vi "grapher.vi"(0 "Eventnum refnum":refnum<vi>, 5 "Frequency refnum":refnum<vi>, 7 "Stop signaller":refnum<class "Signaller.lvclass">, 9 "Polarization refnum":refnum<vi>, 11 "Rate refnum":refnum<vi>) -> ()   [LabVIEW 2018]
uses:
  Motor controller/Signaller/Signaller.lvclass
panel:
  in  "Focus range":dbl=0.1 min=0.001 step=0.1 format="%.3g"
  in  "Focus on current":bool
  in  "Scale for negative":bool
  in  "Scale for positive":bool
  in  "Autoscale polarization":bool=TRUE
  in  "Min polarization":dbl step=0.1 format="%.3g"
  in  "Max polarization":dbl=1.0 step=0.1 format="%.3g"
  in  "Add 1 hour":bool
  in  "1 hour":bool
  in  "30 minutes":bool
  in  "10 minutes":bool
  in  "5 minutes":bool
  in  "1 minute":bool
  in  "Time scale (min)":i64=1 min=1 step=1
  in  "Data output file":path
  out "Data points":i32
  out "Polarization vs frequency":cluster{dbl, dbl}[](graph)
  out "Rate vs time":cluster{"Value":i64, "Value":dbl}[](graph)
  out "Frequency vs time":cluster{"Value":i64, "Value":dbl}[](graph)
  out "Polarization vs time":cluster{i64, dbl}[](graph)
  out "Rate":dbl
  out "Polarization":dbl
  out "Frequency":dbl
  out "Eventnum":i64
  # "Advanced controls"
  # "Graph polarization scale"
  # "Graph time scale"
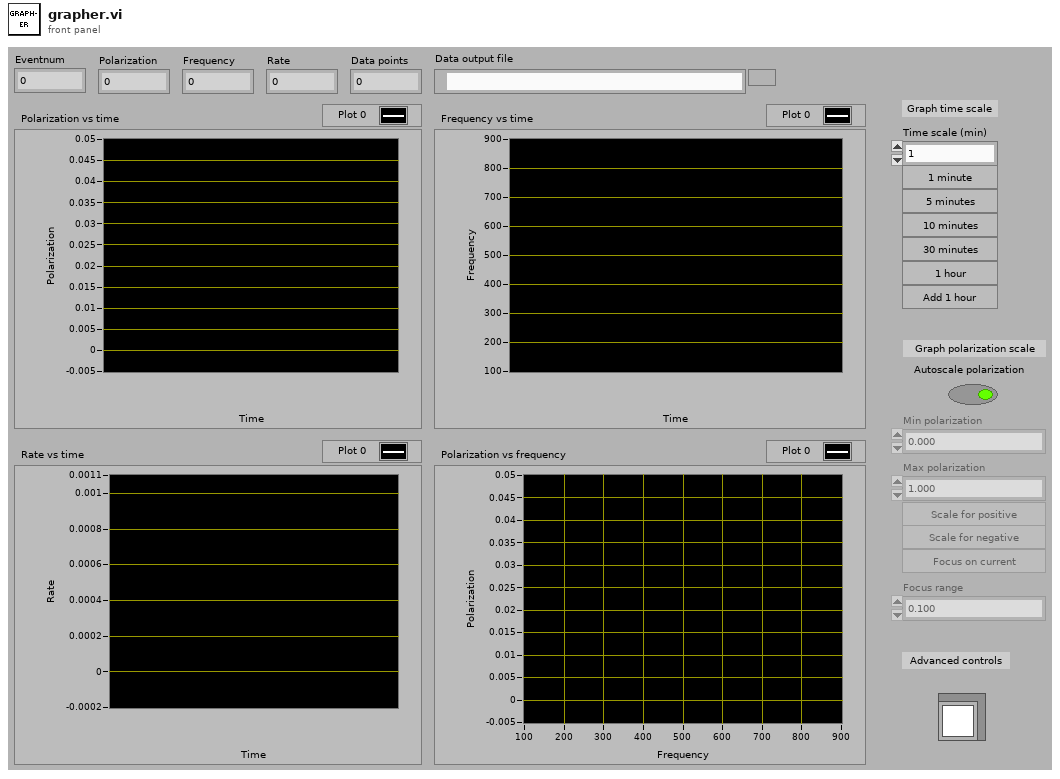
[diagram p1: front panel]
types:
  T1 = typedef "LVRangeTypeDef.ctl" = cluster{"Minimum":dbl, "Maximum":dbl, "Increment":dbl, "Minor Increment":dbl, "Start":dbl}
  T2 = enum8{"Enabled", "Disabled", "Disabled and Grayed Out"}
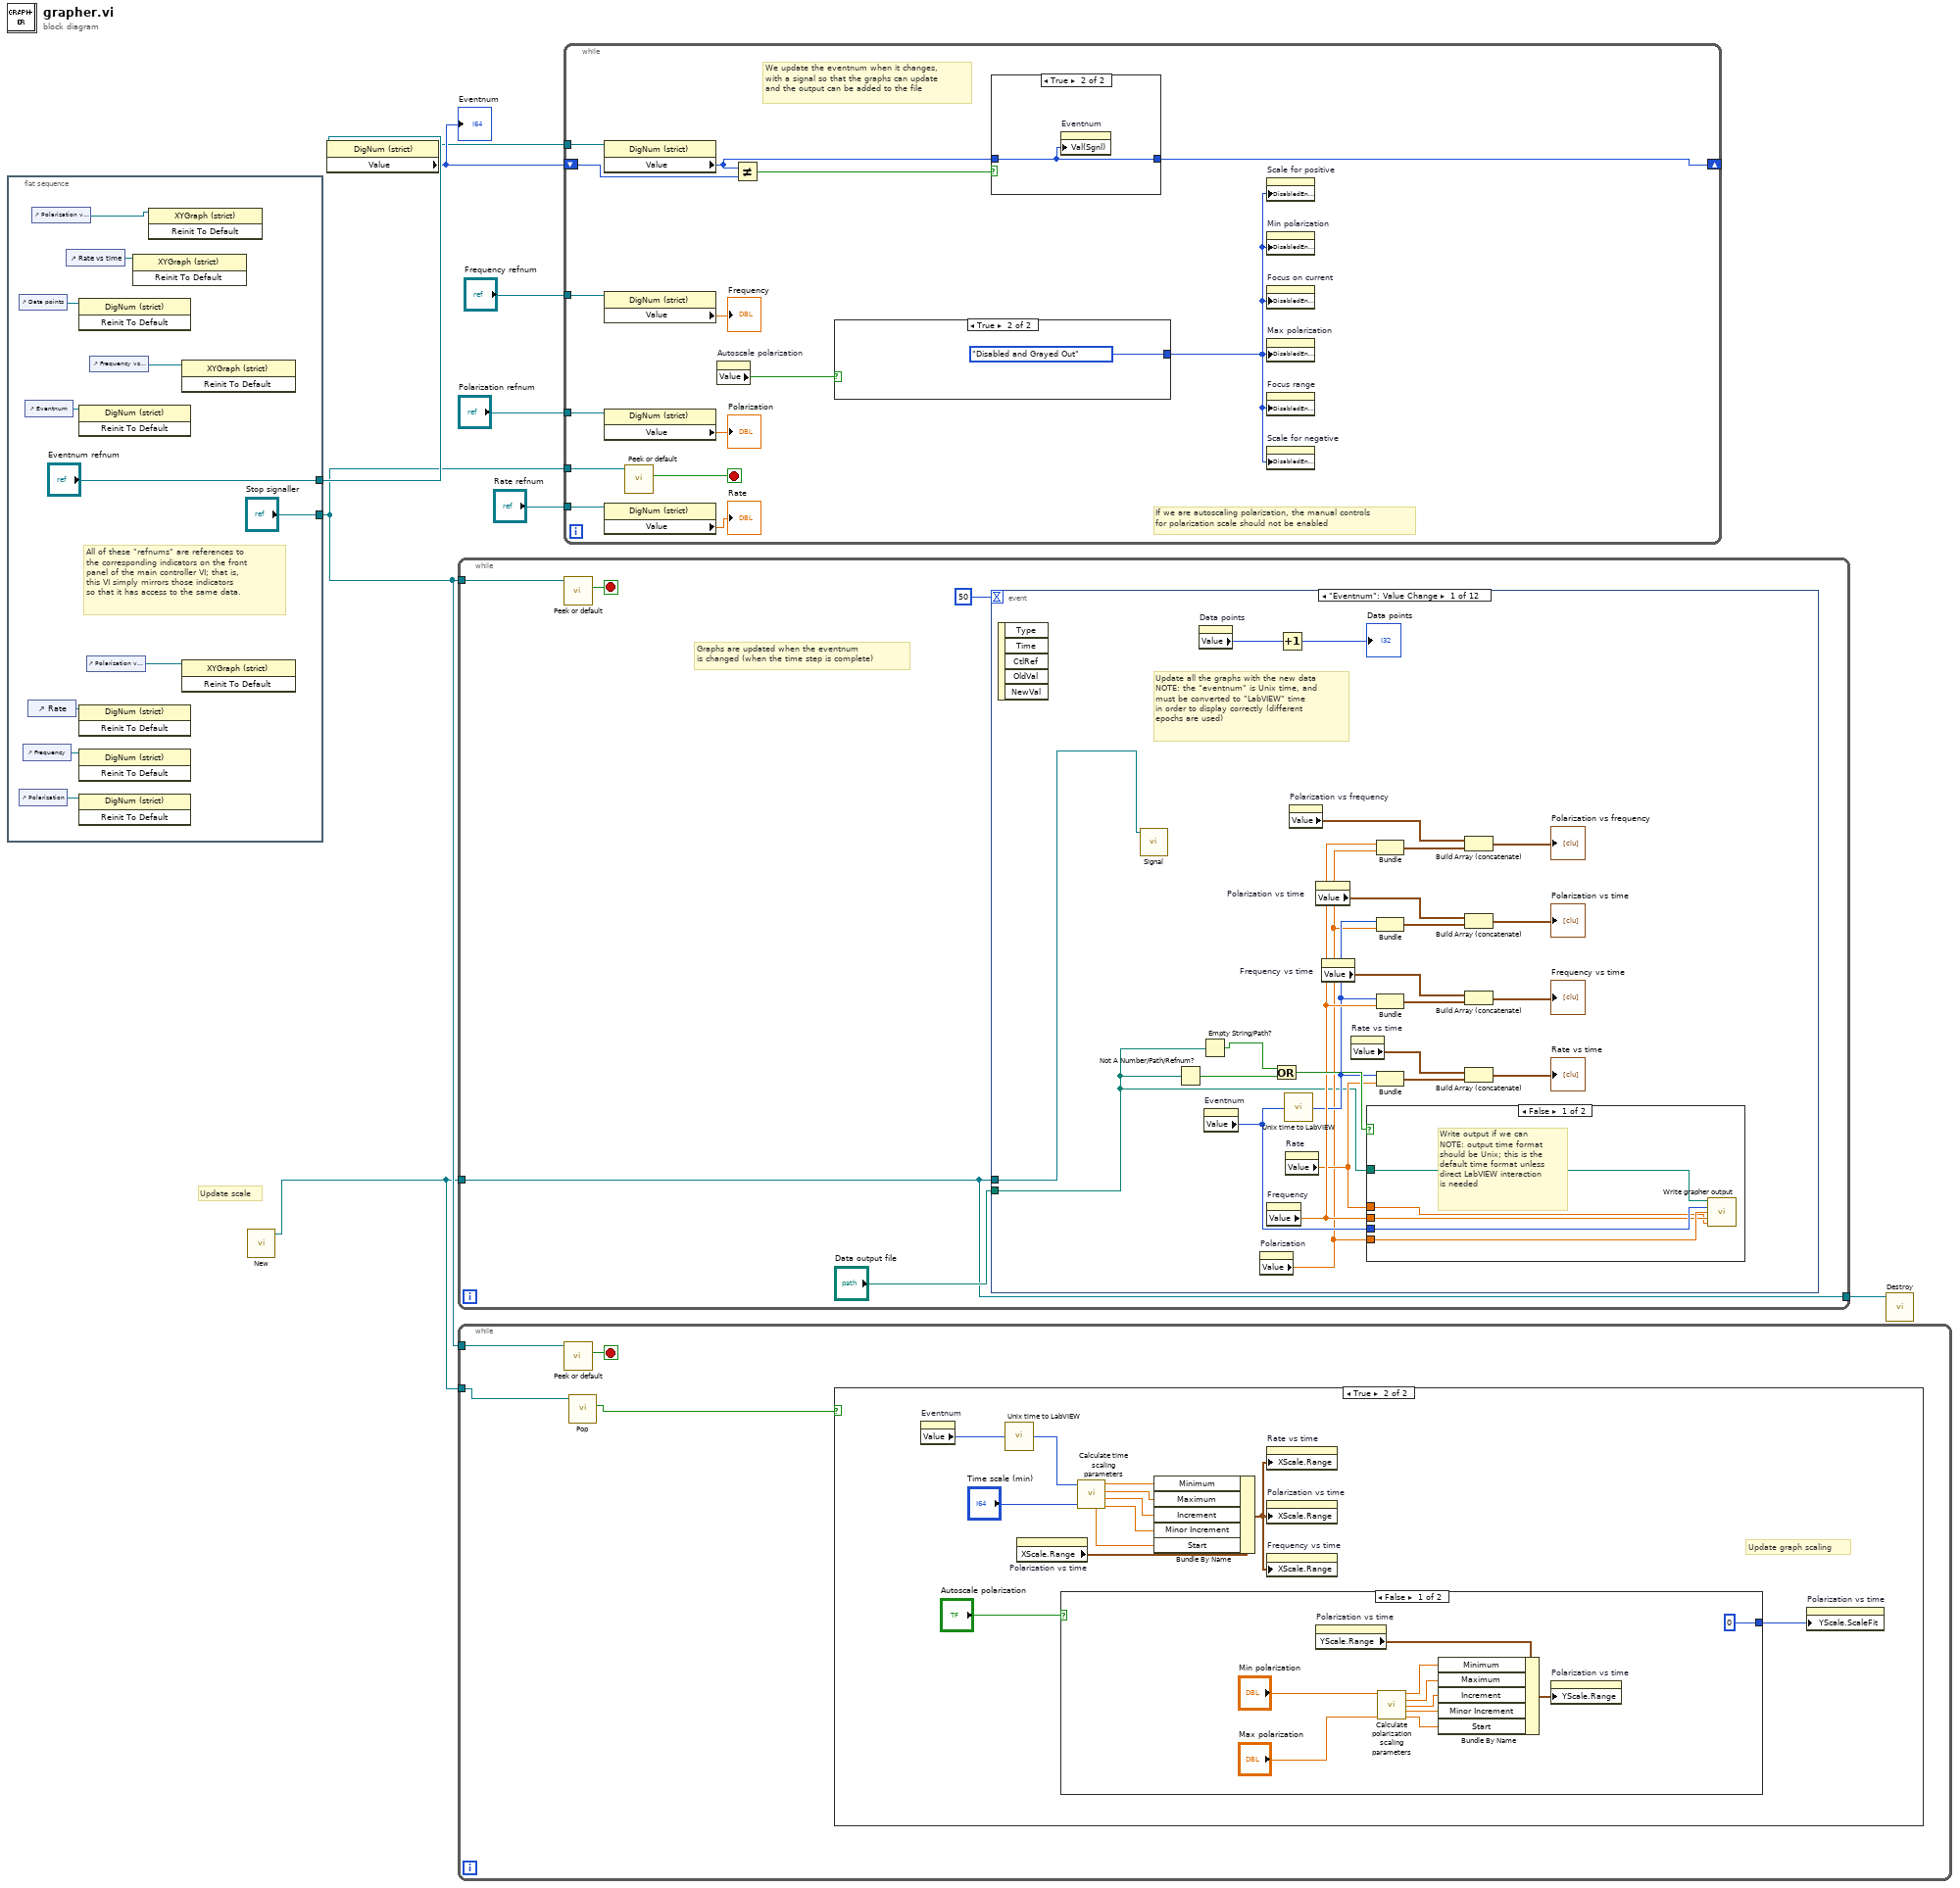
[diagram p0: block diagram]
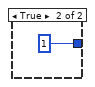
[diagram p3: hidden frame]
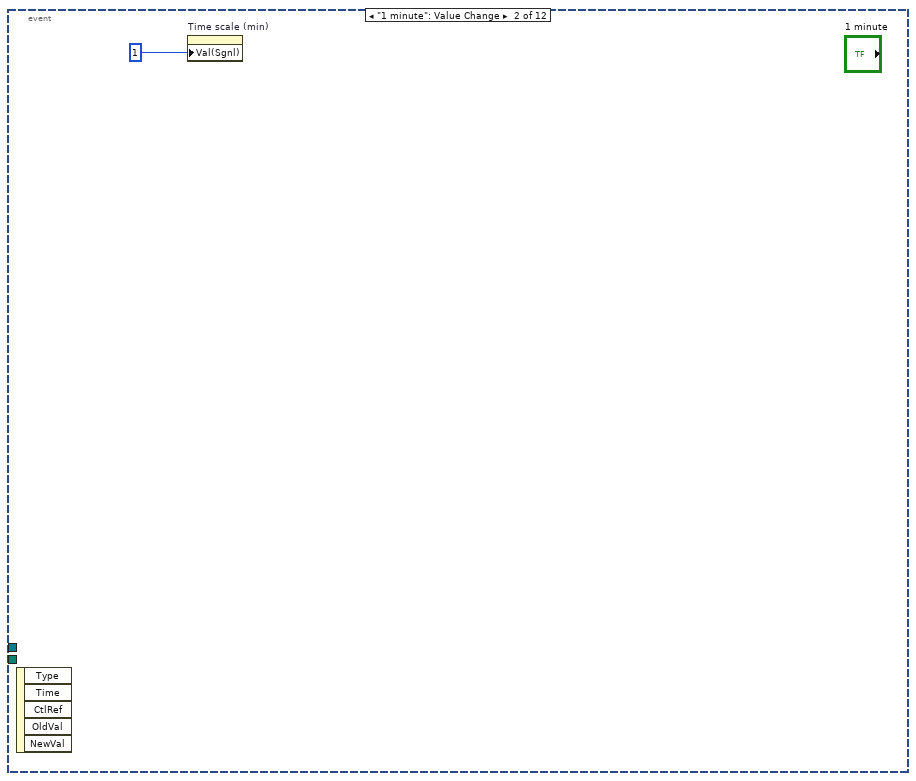
[diagram p5: hidden frame]
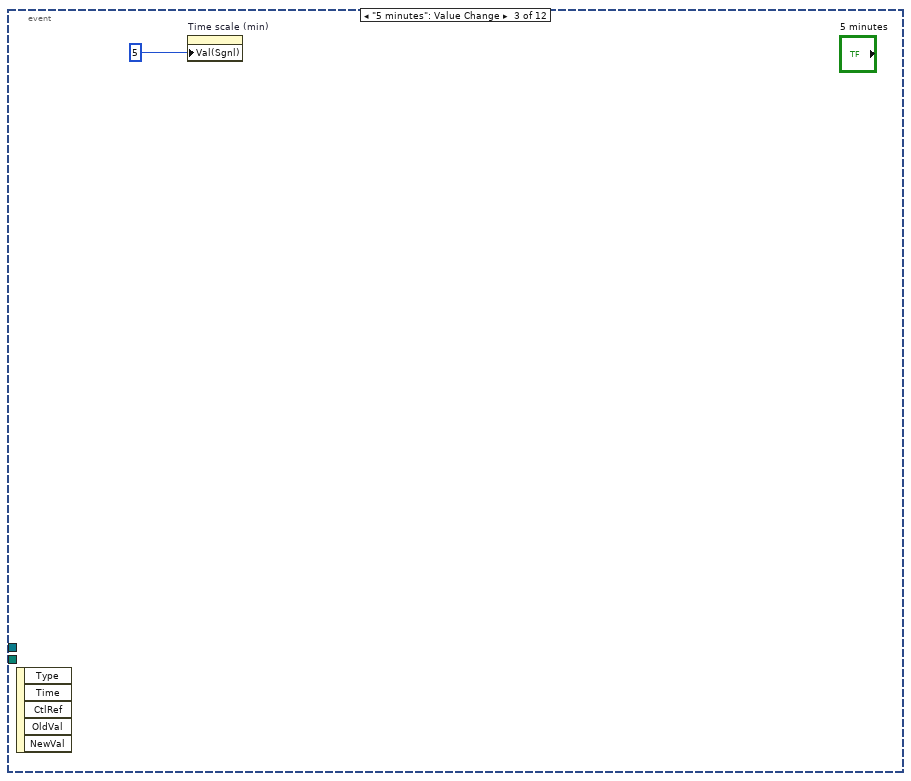
[diagram p6: hidden frame]
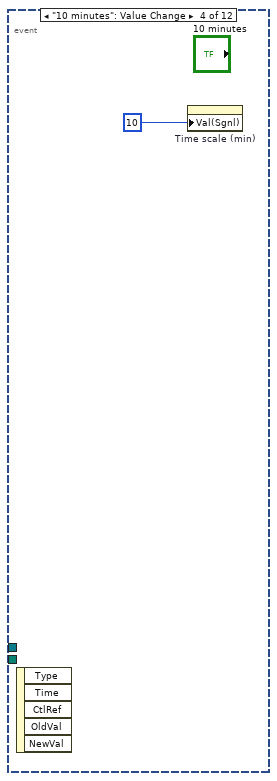
[diagram p7: hidden frame]
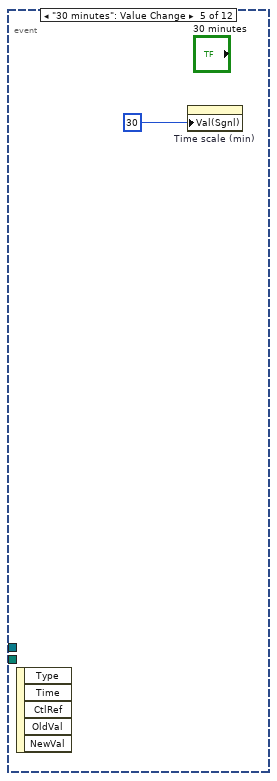
[diagram p8: hidden frame]
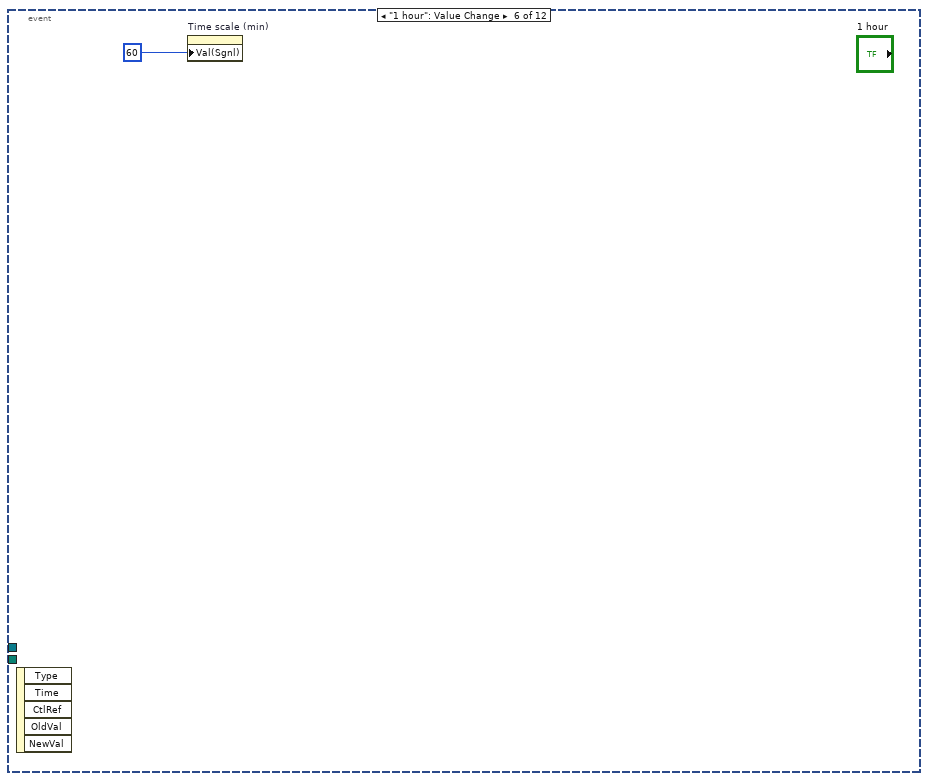
[diagram p9: hidden frame]
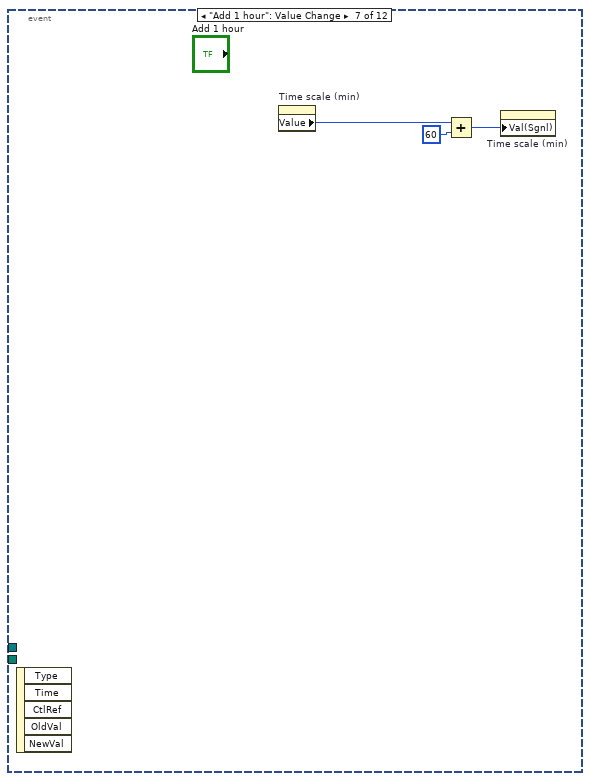
[diagram p10: hidden frame]
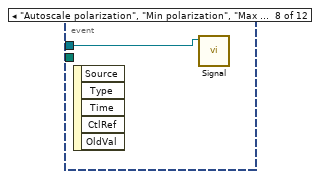
[diagram p11: hidden frame]
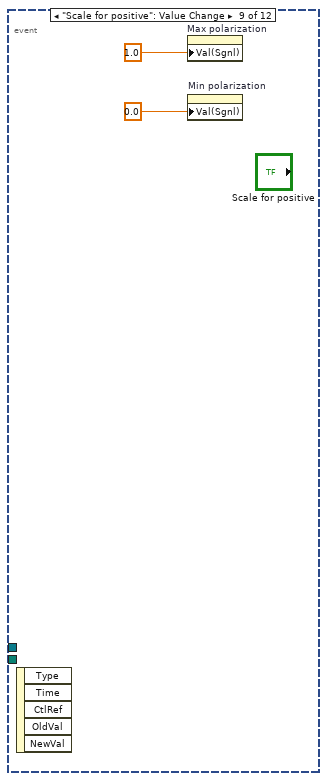
[diagram p12: hidden frame]
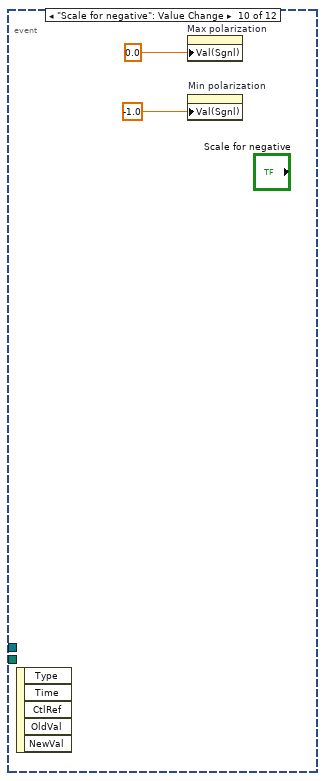
[diagram p13: hidden frame]
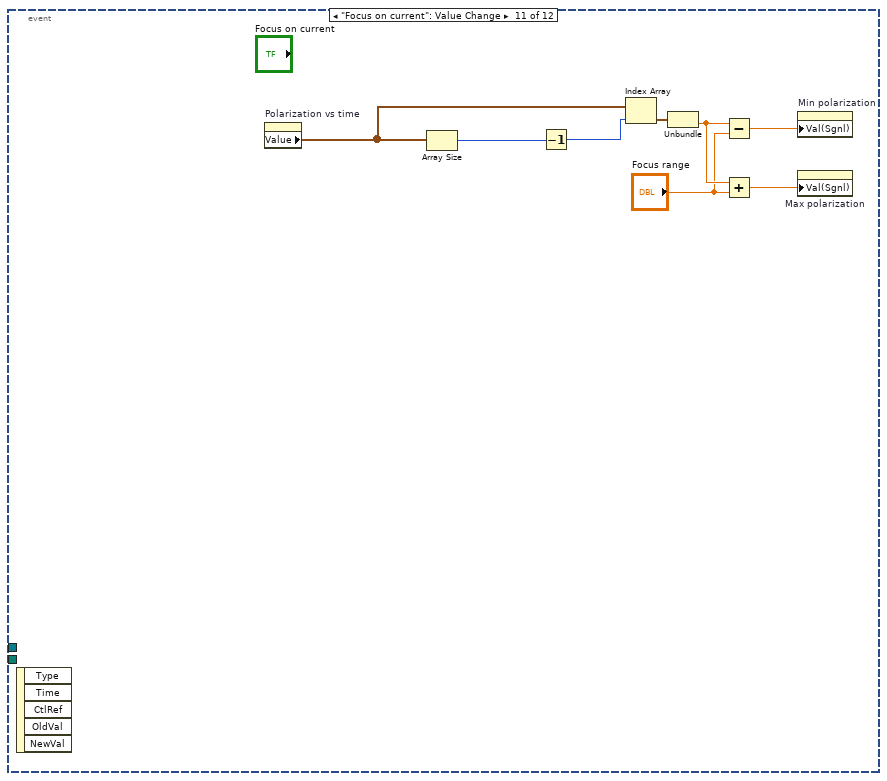
[diagram p14: hidden frame]
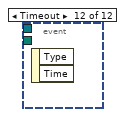
[diagram p15: hidden frame]
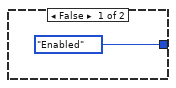
[diagram p16: hidden frame]
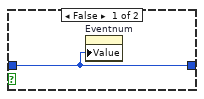
[diagram p17: hidden frame]
diagram:
  # "Update scale"
  n1 = flat-sequence {
    tunnel: ["Eventnum refnum"] -> w6
    tunnel: ["Stop signaller"] -> w2
    frame #0 {
      # "All of these \"refnums\" are references to\nthe corresponding indicators on the front\npanel of the main controller VI; that is,\nthis VI simply mirrors those indicators\nso that it has access to the same data."
      n2 = control-ref of="Data points"() -> (w14:refnum<vi>)
      n3 = control-ref of="Polarization"() -> (w17:refnum<vi>)
      n4 = control-ref of="Frequency"() -> (w16:refnum<vi>)
      n5 = control-ref of="Eventnum"() -> (w18:refnum<vi>)
      n6 = control-ref of="Rate"() -> (w15:refnum<vi>)
      n7 = control-ref of="Polarization vs frequency"() -> (w10:refnum<vi>)
      n8 = control-ref of="Rate vs time"() -> (w11:refnum<vi>)
      n9 = invoke class="DigNum (strict)" method="Reinit To Default"(reference=w14) -> ()  [unwired: 2 in, 3 out]
      n10 = invoke class="DigNum (strict)" method="Reinit To Default"(reference=w18) -> ()  [unwired: 2 in, 3 out]
      n11 = invoke class="DigNum (strict)" method="Reinit To Default"(reference=w15) -> ()  [unwired: 2 in, 3 out]
      n12 = invoke class="DigNum (strict)" method="Reinit To Default"(reference=w16) -> ()  [unwired: 2 in, 3 out]
      n13 = invoke class="DigNum (strict)" method="Reinit To Default"(reference=w17) -> ()  [unwired: 2 in, 3 out]
      n14 = control-ref of="Polarization vs time"() -> (w13:refnum<vi>)
      n15 = control-ref of="Frequency vs time"() -> (w12:refnum<vi>)
      n16 = invoke class="XYGraph (strict)" method="Reinit To Default"(reference=w11) -> ()  [unwired: 2 in, 3 out]
      n17 = invoke class="XYGraph (strict)" method="Reinit To Default"(reference=w10) -> ()  [unwired: 2 in, 3 out]
      n18 = invoke class="XYGraph (strict)" method="Reinit To Default"(reference=w12) -> ()  [unwired: 2 in, 3 out]
      n19 = invoke class="XYGraph (strict)" method="Reinit To Default"(reference=w13) -> ()  [unwired: 2 in, 3 out]
    }
  }
  n20 = call "New.vi"() -> ("Signaller out"=w1:refnum<class "Signaller.lvclass">)  [unwired: 11 in]
  n21 = property class="DigNum (strict)"(reference=w6) -> (reference out=w4:refnum<vi>, "Value"=w5:i64)  [unwired: 1 in, 1 out]
  "Eventnum" <- w5
  n22 = while {
    tunnel: w2 -> [w23]
    tunnel: w1 -> [w21]
    tunnel: [w21] -> w3
    stop <- w22 stop-if-true
    # "Graphs are updated when the eventnum\nis changed (when the time step is complete)"
    n23 = call "Peek or default.vi"("Signaller in"=w23) -> ("Has signal?"=w22:bool)  [unwired: 8 in, 2 out]
    n24 = event shown="[0] \"Eventnum\": Value Change" {
      selector: _ -> [_ _ _ _ _ _ _ _ _ _ _ _]
      dyn-events: _ -> [_ _ _ _ _ _ _ _ _ _ _ _]
      timeout: 50 -> [_ _ _ _ _ _ _ _ _ _ _ _]
      tunnel: "Data output file" -> [w27 _ _ _ _ _ _ _ _ _ _ _]
      tunnel: w21 -> [w28 _ _ _ _ _ _ w63 _ _ _ _]
      event "Eventnum": Value Change {
        # "Update all the graphs with the new data\nNOTE: the \"eventnum\" is Unix time, and\nmust be converted to \"LabVIEW\" time\nin order to display correctly (different\nepochs are used)"
        n25 = event-data() -> ()  [unwired: 1 in, 5 out]
        n26 = call "Signal.vi"("Signaller in"=w28) -> ()  [unwired: 9 in, 2 out]
        n27 = Not A Number/Path/Refnum?(number/path/refnum=w27) -> (NaN/Path/Refnum?=w45:bool)
        n28 = property on="Data points" class="DigNum (strict)"() -> ("Value"=w30:i32)  [unwired: 2 in, 2 out]
        n29 = Empty String/Path?(string/path=w27) -> (empty?=w26:bool)
        n30 = property on="Eventnum" class="DigNum (strict)"() -> ("Value"=w41:i64)  [unwired: 2 in, 2 out]
        n31 = property on="Polarization" class="DigNum (strict)"() -> ("Value"=w29:dbl)  [unwired: 2 in, 2 out]
        n32 = property on="Frequency" class="DigNum (strict)"() -> ("Value"=w43:dbl)  [unwired: 2 in, 2 out]
        n33 = Or(x=w26, y=w45) -> (x .or. y?=w44:bool)
        n34 = Increment(x=w30) -> (x+1=→"Data points":i32)
        n35 = call "Unix time to LabVIEW.vi"("Unix time"=w41) -> ("LabVIEW time"=w40:i64)
        n36 = property on="Rate" class="DigNum (strict)"() -> ("Value"=w42:dbl)  [unwired: 2 in, 2 out]
        n37 = property on="Polarization vs frequency" class="XYGraph (strict)"() -> ("Value"=w32:cluster{dbl, dbl}[])  [unwired: 2 in, 2 out]
        n38 = property on="Polarization vs time" class="XYGraph (strict)"() -> ("Value"=w35:cluster{i64, dbl}[])  [unwired: 2 in, 2 out]
        n39 = property on="Frequency vs time" class="XYGraph (strict)"() -> ("Value"=w34:cluster{"Value":i64, "Value":dbl}[])  [unwired: 2 in, 2 out]
        n40 = property on="Rate vs time" class="XYGraph (strict)"() -> ("Value"=w33:cluster{"Value":i64, "Value":dbl}[])  [unwired: 2 in, 2 out]
        n41 = case shown="False" w44 {
          tunnel: w27 -> [w54 _]
          tunnel: w41 -> [w53 _]
          tunnel: w29 -> [w52 _]
          tunnel: w43 -> [w51 _]
          tunnel: w42 -> [w50 _]
          frame False {
            # "Write output if we can\nNOTE: output time format\nshould be Unix; this is the\ndefault time format unless\ndirect LabVIEW interaction\nis needed"
            n42 = call "Write grapher output.vi"("Data output file"=w54, "Time"=w53, "Polarization"=w52, "Frequency"=w51, "Rate"=w50) -> ()  [unwired: 11 in]
          }
          frame True {
          }
        }
        n43 = Bundle("Value"=w43, "Value"=w29) -> (w48:cluster{"Value":dbl, "Value":dbl})  [unwired: 1 in]
        n44 = Bundle("LabVIEW time"=w40, "Value"=w29) -> (w46:cluster{"LabVIEW time":i64, "Value":dbl})  [unwired: 1 in]
        n45 = Bundle("LabVIEW time"=w40, "Value"=w43) -> (w47:cluster{"LabVIEW time":i64, "Value":dbl})  [unwired: 1 in]
        n46 = Bundle("LabVIEW time"=w40, "Value"=w42) -> (w49:cluster{"LabVIEW time":i64, "Value":dbl})  [unwired: 1 in]
        n47 = Build Array (concatenate)(w32, w48) -> (→"Polarization vs frequency":cluster{"Value":dbl, "Value":dbl}[])
        n48 = Build Array (concatenate)(w35, w46) -> (→"Polarization vs time":cluster{"LabVIEW time":i64, "Value":dbl}[])
        n49 = Build Array (concatenate)(w34, w47) -> (→"Frequency vs time":cluster{"LabVIEW time":i64, "Value":dbl}[])
        n50 = Build Array (concatenate)(w33, w49) -> (→"Rate vs time":cluster{"LabVIEW time":i64, "Value":dbl}[])
      }
      event "1 minute": Value Change {
        n51 = event-data() -> ()  [unwired: 1 in, 5 out]
        n52 = property on="Time scale (min)" class="DigNum (strict)"("Val(Sgnl)"=i64 1 ("Value (Signaling)")) -> ()  [unwired: 2 in, 2 out]
      }
      event "5 minutes": Value Change {
        n53 = event-data() -> ()  [unwired: 1 in, 5 out]
        n54 = property on="Time scale (min)" class="DigNum (strict)"("Val(Sgnl)"=i64 5 ("Value (Signaling)")) -> ()  [unwired: 2 in, 2 out]
      }
      event "10 minutes": Value Change {
        n55 = event-data() -> ()  [unwired: 1 in, 5 out]
        n56 = property on="Time scale (min)" class="DigNum (strict)"("Val(Sgnl)"=i64 10 ("Value (Signaling)")) -> ()  [unwired: 2 in, 2 out]
      }
      event "30 minutes": Value Change {
        n57 = event-data() -> ()  [unwired: 1 in, 5 out]
        n58 = property on="Time scale (min)" class="DigNum (strict)"("Val(Sgnl)"=i64 30 ("Value (Signaling)")) -> ()  [unwired: 2 in, 2 out]
      }
      event "1 hour": Value Change {
        n59 = event-data() -> ()  [unwired: 1 in, 5 out]
        n60 = property on="Time scale (min)" class="DigNum (strict)"("Val(Sgnl)"=i64 60 ("Value (Signaling)")) -> ()  [unwired: 2 in, 2 out]
      }
      event "Add 1 hour": Value Change {
        n61 = event-data() -> ()  [unwired: 1 in, 5 out]
        n62 = property on="Time scale (min)" class="DigNum (strict)"() -> ("Value"=w62:i64)  [unwired: 2 in, 2 out]
        n63 = Add(x=w62, y=i64 60) -> (x+y=w60:i64)
        n64 = property on="Time scale (min)" class="DigNum (strict)"("Val(Sgnl)"=w60) -> ()  [unwired: 2 in, 2 out]
      }
      event "Autoscale polarization", "Min polarization", "Max polarization", "Time scale (min)": Value Change {
        n65 = event-data() -> ()  [unwired: 1 in, 5 out]
        n66 = call "Signal.vi"("Signaller in"=w63) -> ()  [unwired: 9 in, 2 out]
      }
      event "Scale for positive": Value Change {
        n67 = event-data() -> ()  [unwired: 1 in, 5 out]
        n68 = property on="Max polarization" class="DigNum (strict)"("Val(Sgnl)"=1.0 ("Value (Signaling)")) -> ()  [unwired: 2 in, 2 out]
        n69 = property on="Min polarization" class="DigNum (strict)"("Val(Sgnl)"=0.0 ("Value (Signaling)")) -> ()  [unwired: 2 in, 2 out]
      }
      event "Scale for negative": Value Change {
        n70 = event-data() -> ()  [unwired: 1 in, 5 out]
        n71 = property on="Max polarization" class="DigNum (strict)"("Val(Sgnl)"=0.0 ("Value (Signaling)")) -> ()  [unwired: 2 in, 2 out]
        n72 = property on="Min polarization" class="DigNum (strict)"("Val(Sgnl)"=-1.0 ("Value (Signaling)")) -> ()  [unwired: 2 in, 2 out]
      }
      event "Focus on current": Value Change {
        n73 = event-data() -> ()  [unwired: 1 in, 5 out]
        n74 = property on="Polarization vs time" class="XYGraph (strict)"() -> ("Value"=w75:cluster{i64, dbl}[])  [unwired: 2 in, 2 out]
        n75 = Array Size(array=w75) -> (size(s)=w74:i32)
        n76 = Decrement(x=w74) -> (x-1=w73:i32)
        n77 = Index Array(array=w75, index=w73) -> (element=w72:cluster{i64, dbl})
        n78 = Unbundle(w72) -> (w69:dbl)  [unwired: 1 out]
        n79 = Subtract(x=w69, y="Focus range") -> (x-y=w70:dbl)
        n80 = Add(x=w69, y="Focus range") -> (x+y=w71:dbl)
        n81 = property on="Min polarization" class="DigNum (strict)"("Val(Sgnl)"=w70) -> ()  [unwired: 2 in, 2 out]
        n82 = property on="Max polarization" class="DigNum (strict)"("Val(Sgnl)"=w71) -> ()  [unwired: 2 in, 2 out]
      }
      event Timeout {
        n83 = event-data() -> ()  [unwired: 1 in, 2 out]
      }
    }
  }
  n84 = while {
    tunnel: w1 -> [w77]
    tunnel: w2 -> [w79]
    stop <- w78 stop-if-true
    n85 = call "Peek or default.vi"("Signaller in"=w79) -> ("Has signal?"=w78:bool)  [unwired: 8 in, 2 out]
    n86 = call "Pop.vi"("Signaller in"=w77) -> ("Has signal"=w76:bool)  [unwired: 8 in, 2 out]
    n87 = case shown="True" w76 {
      frame False {
      }
      frame True {
        # "Update graph scaling"
        n88 = property on="Eventnum" class="DigNum (strict)"() -> ("Value"=w83:i64)  [unwired: 2 in, 2 out]
        n89 = call "Unix time to LabVIEW.vi"("Unix time"=w83) -> ("LabVIEW time"=w82:i64)
        n90 = property on="Polarization vs time" class="XYGraph (strict)"() -> ("XScale.Range"=w91:T1)  [unwired: 2 in, 2 out]
        n91 = case shown="False" "Autoscale polarization" {
          tunnel: [u8 0 ("Y Scale.Scale Fit") u8 1 ("Y Scale.Scale Fit")] -> w80
          frame False {
            n92 = property on="Polarization vs time" class="XYGraph (strict)"() -> ("YScale.Range"=w99:T1)  [unwired: 2 in, 2 out]
            n93 = call "Calculate polarization scaling parameters.vi"("Min polarization"="Min polarization", "Max polarization"="Max polarization") -> ("Minimum"=w97:dbl, "Maximum"=w96:dbl, "Increment"=w95:dbl, "Minor increment"=w94:dbl, "Start"=w93:dbl)  [unwired: 9 in]
            n94 = Bundle By Name(cluster=w99, "Minimum"=w97, "Maximum"=w96, "Increment"=w95, "Minor Increment"=w94, "Start"=w93) -> (w98:T1)
            n95 = property on="Polarization vs time" class="XYGraph (strict)"("YScale.Range"=w98) -> ()  [unwired: 2 in, 2 out]
          }
          frame True {
          }
        }
        n96 = call "Calculate time scaling parameters.vi"("Time"=w82, "Time scale (minutes)"="Time scale (min)") -> ("Minimum"=w88:dbl, "Maximum"=w87:dbl, "Increment"=w86:dbl, "Minor increment"=w85:dbl, "Start"=w90:dbl)  [unwired: 1 in]
        n97 = Bundle By Name(cluster=w91, "Minimum"=w88, "Maximum"=w87, "Increment"=w86, "Minor Increment"=w85, "Start"=w90) -> (w89:T1)
        n98 = property on="Rate vs time" class="XYGraph (strict)"("XScale.Range"=w89) -> ()  [unwired: 2 in, 2 out]
        n99 = property on="Polarization vs time" class="XYGraph (strict)"("XScale.Range"=w89) -> ()  [unwired: 2 in, 2 out]
        n100 = property on="Frequency vs time" class="XYGraph (strict)"("XScale.Range"=w89) -> ()  [unwired: 2 in, 2 out]
        n101 = property on="Polarization vs time" class="XYGraph (strict)"("YScale.ScaleFit"=w80) -> ()  [unwired: 2 in, 2 out]
      }
    }
  }
  n102 = while {
    tunnel: "Polarization refnum" -> [w117]
    tunnel: "Frequency refnum" -> [w116]
    tunnel: w4 -> [w115]
    tunnel: "Rate refnum" -> [w114]
    shift-right: [w110] -> _
    shift-left: w5 -> [w111]
    tunnel: w2 -> [w106]
    stop <- w105 stop-if-true
    # "We update the eventnum when it changes,\nwith a signal so that the graphs can update\nand the output can be added to the file"
    # "If we are autoscaling polarization, the manual controls\nfor polarization scale should not be enabled"
    n103 = property class="DigNum (strict)"(reference=w115) -> ("Value"=w112:i64)  [unwired: 1 in, 2 out]
    n104 = property class="DigNum (strict)"(reference=w116) -> ("Value"=→"Frequency":dbl)  [unwired: 1 in, 2 out]
    n105 = property class="DigNum (strict)"(reference=w117) -> ("Value"=→"Polarization":dbl)  [unwired: 1 in, 2 out]
    n106 = property class="DigNum (strict)"(reference=w114) -> ("Value"=→"Rate":dbl)  [unwired: 1 in, 2 out]
    n107 = call "Peek or default.vi"("Signaller in"=w106) -> ("Has signal?"=w105:bool)  [unwired: 8 in, 2 out]
    n108 = property on="Autoscale polarization" class="Bool (strict)"() -> ("Value"=w104:bool)  [unwired: 2 in, 2 out]
    n109 = Not Equal?(x=w112, y=w111) -> (x != y?=w113:bool)
    n110 = case shown="True" w104 {
      tunnel: [T2."Enabled" ("Disabled") T2."Disabled and Grayed Out" ("Disabled")] -> w103
      frame False {
      }
      frame True {
      }
    }
    n111 = case shown="True" w113 {
      tunnel: w112 -> [w120 w121]
      tunnel: [w120 w121] -> w110
      frame False {
        n112 = property on="Eventnum" class="DigNum (strict)"("Value"=w120) -> ()  [unwired: 2 in, 2 out]
      }
      frame True {
        n113 = property on="Eventnum" class="DigNum (strict)"("Val(Sgnl)"=w121) -> ()  [unwired: 2 in, 2 out]
      }
    }
    n114 = property on="Scale for positive" class="Bool"("DisabledEnum"=w103) -> ()  [unwired: 2 in, 2 out]
    n115 = property on="Min polarization" class="DigNum (strict)"("DisabledEnum"=w103) -> ()  [unwired: 2 in, 2 out]
    n116 = property on="Focus on current" class="Bool"("DisabledEnum"=w103) -> ()  [unwired: 2 in, 2 out]
    n117 = property on="Max polarization" class="DigNum (strict)"("DisabledEnum"=w103) -> ()  [unwired: 2 in, 2 out]
    n118 = property on="Focus range" class="DigNum (strict)"("DisabledEnum"=w103) -> ()  [unwired: 2 in, 2 out]
    n119 = property on="Scale for negative" class="Bool"("DisabledEnum"=w103) -> ()  [unwired: 2 in, 2 out]
  }
  n120 = call "Destroy.vi"("Signaller in"=w3) -> ()  [unwired: 10 in, 1 out]
